vi "ips120 ramp to field.vi"(8 "error in (no error)":errorcluster, 10 "target field (T)":dbl, 11 "VISA resource name":refnum<visa-resource-name>) -> (0 "error out":errorcluster, 3 "VISA resource name 2":refnum<visa-resource-name>)   [LabVIEW 2013]
panel:
  # "Ramps the magnet to the specified field.\n\nThis VI also verifies that the switch heater is turned on.\nThis VI is blocking, i.e. it waits until the ramp is completed."
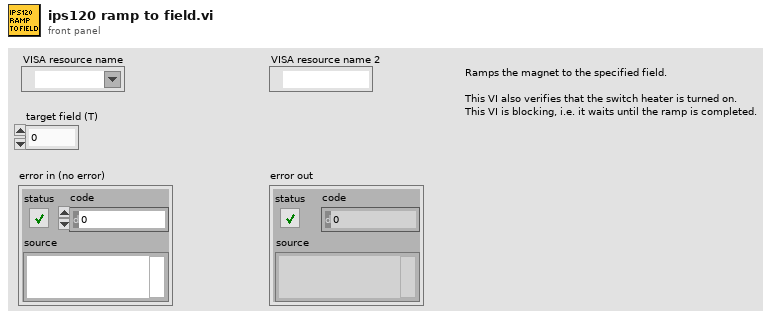
[diagram p1: front panel]
types:
  T1 = enum16{"hold", "to set point", "to zero", "clamp"}
  T2 = enum16{"heater off", "heater on psu=magnet", "heater on, no checks"}
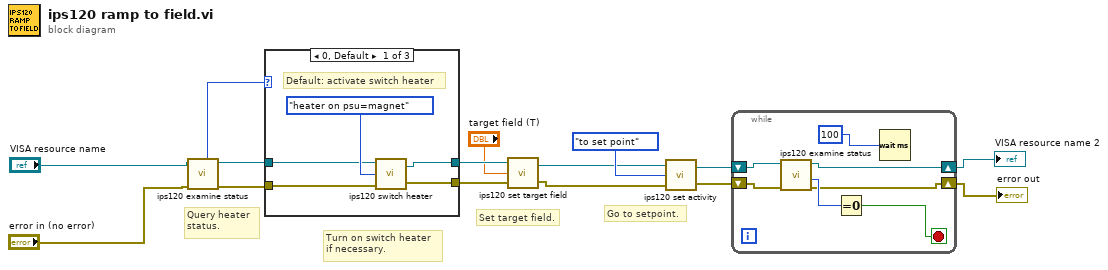
[diagram p0: block diagram]
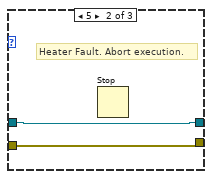
[diagram p2: hidden frame]
diagram:
  # "Set target field."
  # "Go to setpoint."
  # "Turn on switch heater\nif necessary."
  # "Query heater \nstatus."
  n1 = call "ips120 examine status.vi"("error in (no error)"="error in (no error)", "VISA resource name"="VISA resource name") -> ("error out"=w13:errorcluster, "VISA resource name 2"=w14:refnum<visa-resource-name>, "switch heater status"=w15:i8)  [unwired: 1 in, 6 out]
  n2 = case shown="0, Default" w15 {
    tunnel: w14 -> [w19 w22 w24]
    tunnel: w13 -> [w18 w21 w23]
    tunnel: [w17 w22 w24] -> w7
    tunnel: [w16 w21 w23] -> w6
    frame 0, Default {
      # "Default: activate switch heater"
      n3 = call "ips120 switch heater.vi"("error in (no error)"=w18, "switch heater status"=T2."heater on psu=magnet", "VISA resource name"=w19) -> ("error out"=w16:errorcluster, "VISA resource name 2"=w17:refnum<visa-resource-name>)  [unwired: 1 in]
    }
    frame 5 {
      # "Heater Fault. Abort execution."
      n4 = Stop() -> ()  [unwired: 1 in]
    }
    frame 1 {
      # "1 == Heater is on.\nNo action needed."
    }
  }
  n5 = call "ips120 set target field.vi"("error in (no error)"=w6, "target field (T)"="target field (T)", "VISA resource name"=w7) -> ("error out"=w5:errorcluster, "VISA resource name"=w4:refnum<visa-resource-name>)
  n6 = call "ips120 set activity.vi"("error in (no error)"=w5, "activity"=T1."to set point", "VISA resource name"=w4) -> ("error out"=w11:errorcluster, "VISA resource name 2"=w10:refnum<visa-resource-name>)
  n7 = while {
    shift-right: [w27] -> w9
    shift-left: w11 -> [w30]
    shift-right: [w26] -> w8
    shift-left: w10 -> [w31]
    stop <- w28 stop-if-true
    n8 = call "ips120 examine status.vi"("error in (no error)"=w30, "VISA resource name"=w31) -> ("error out"=w27:errorcluster, "sweep status"=w29:i8, "VISA resource name 2"=w26:refnum<visa-resource-name>)  [unwired: 1 in, 6 out]
    n9 = Equal To 0?(x=w29) -> (x = 0?=w28:bool)
    n10 = Wait (ms)(milliseconds to wait=100) -> ()  [unwired: 1 out]
  }
  "error out" <- w9
  "VISA resource name 2" <- w8
